vi "write_log_metadata.vi"(8 "error in (no error)":errorcluster, 10 "data":variant, 11 "pcfs_hdf5_log in":refnum<class "pcfs_hdf5_log.lvclass">) -> (0 "error out":errorcluster, 3 "pcfs_hdf5_log out":refnum<class "pcfs_hdf5_log.lvclass">)   [LabVIEW 2015, in "pcfs_hdf5_log.lvclass"]
uses:
  pcfs_hdf5_log.lvclass
  pcfs_settings.ctl
  Scan/scan_record.ctl
  Detector_Class/Picoquant/Hydraharp/hydraharp_panel/hpanel_acq_modes.ctl
  pcfs_hdf5_log.lvclass/pcfs_hdf5_log.ctl
  <vilib>/UPVI/lvhdf5/attribute.llb/LVH5A Operation.ctl
  <vilib>/UPVI/lvhdf5/attribute.llb/Simple H5Awrite (Variant).vi
  <vilib>/UPVI/lvhdf5/attribute.llb/Simple H5Awrite.xnode
  <vilib>/UPVI/lvhdf5/library.llb/HDF5 Ref.ctl
  Detector_Class/Picoquant/Hydraharp/hdf5_photon_record_logger/hdf5_photon_record_log.lvclass
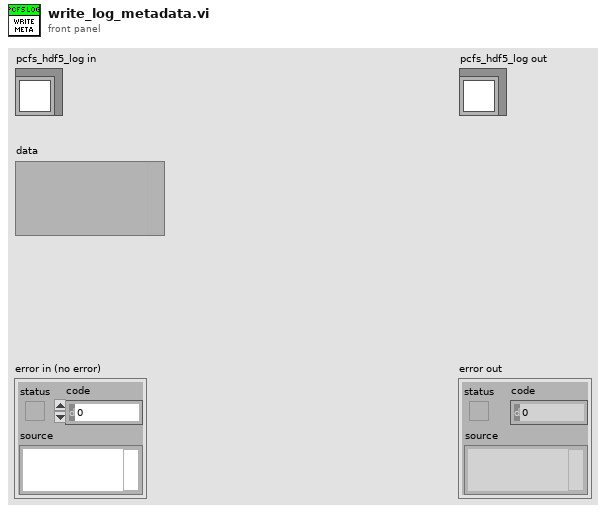
[diagram p1: front panel]
types:
  T1 = typedef "pcfs_settings.ctl" = cluster{"Center Pos. (mm)":dbl, "Increment (mm)":dbl, "Steps":dbl, "Dither Dist (nm)":dbl, "Dither Period (s)":dbl, "Cycles":dbl, "Record Type":T2, "Save Path":path, "Stage Number":enum16{"1", "2"}, "File Notes":string, "Mode":T3, "overwrite":bool, "custom_path":bool, "custom_positions":dbl[]}
  T2 = typedef "scan_record.ctl" = enum16{"hdf5", "legacy", "None"}
  T3 = typedef "hpanel_acq_modes.ctl" = u16
  T4 = typedef "LVH5A Operation.ctl" = enum16{"open", "replace", "create", "open or create", "create or replace", "create or replace with confirmation"}
  T5 = typedef "HDF5 Ref.ctl" = refnum<k1>
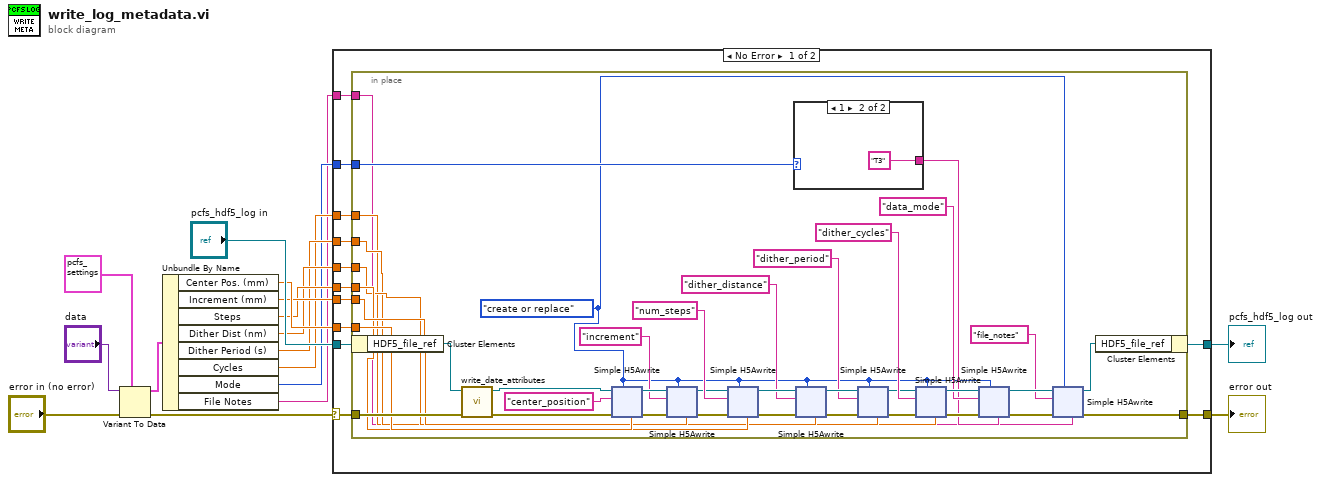
[diagram p0: block diagram]
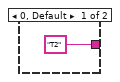
[diagram p2: hidden frame]
diagram:
  n1 = Variant To Data(error in="error in (no error)", type=T1 {"Center Pos. (mm)"=0.0, "Increment (mm)"=10.0, "Steps"=10.0, "Dither Dist (nm)"=10.0, "Dither Period (s)"=10.0, "Cycles"=10.0, "Record Type"=enum."hdf5", "Save Path"=path "C:/Users/bspoka/Desktop/test_pcfs", "Stage Number"=enum."1", "File Notes"="", "Mode"=2, "overwrite"=FALSE, "custom_path"=FALSE, "custom_positions"=[]} ("pcfs_settings"), Variant="data") -> (data=w11:T1, error out=w14:errorcluster)
  n2 = Unbundle By Name(w11) -> ("Center Pos. (mm)"=w10:dbl, "Increment (mm)"=w9:dbl, "Steps"=w8:dbl, "Dither Dist (nm)"=w7:dbl, "Dither Period (s)"=w6:dbl, "Cycles"=w5:dbl, "Mode"=w4:T3, "File Notes"=w3:string)
  n3 = case shown="No Error" w14 {
    selector: w14 -> [w27 w189]
    tunnel: "pcfs_hdf5_log in" -> [w28 w190]
    tunnel: w10 -> [w26 _]
    tunnel: w9 -> [w25 _]
    tunnel: w8 -> [w24 _]
    tunnel: w7 -> [w23 _]
    tunnel: w6 -> [w22 _]
    tunnel: w5 -> [w21 _]
    tunnel: w4 -> [w20 _]
    tunnel: w3 -> [w19 _]
    tunnel: [w18 w190] -> w2
    tunnel: [w17 w189] -> w1
    frame No Error {
      n4 = in-place {
        in-place-border: w27 -> [w65]
        in-place-border: w26 -> [w61]
        in-place-border: w25 -> [w57]
        in-place-border: w24 -> [w54]
        in-place-border: w23 -> [w49]
        in-place-border: w22 -> [w45]
        in-place-border: w21 -> [w42]
        in-place-border: w20 -> [w37]
        in-place-border: w19 -> [w32]
        in-place-border: [w29] -> w17
        w31 = LVH5A_Operation."create or replace" ("operation (open or create)")
        n5 = in-place-cluster #1(w28) -> ("HDF5_file_ref"=w66:T5)
        n6 = call "write_date_attributes.vi"("error in (no error)"=w65, "HDF5 Ref"=w66) -> ("error out"=w64:errorcluster, "HDF5 Ref out"=w63:T5)  [unwired: 8 in]
        n7 = xnode "Simple H5Awrite"("HDF5 Ref"=w63, "Name"="center_position", "error in (no error)"=w64, "operation (open or create)"=w31, "Value"=w61) -> ("HDF5 Ref out"=w59:T5, "error out"=w60:errorcluster)
        n8 = xnode "Simple H5Awrite"("HDF5 Ref"=w59, "Name"="increment", "error in (no error)"=w60, "operation (open or create)"=w31, "Value"=w57) -> ("HDF5 Ref out"=w55:T5, "error out"=w53:errorcluster)
        n9 = xnode "Simple H5Awrite"("HDF5 Ref"=w55, "Name"="num_steps", "error in (no error)"=w53, "operation (open or create)"=w31, "Value"=w54) -> ("HDF5 Ref out"=w51:T5, "error out"=w52:errorcluster)
        n10 = case shown="1" w37 {
          tunnel: ["T2" "T3"] -> w36
          frame 0, Default {
          }
          frame 1 {
          }
        }
        n11 = xnode "Simple H5Awrite"("HDF5 Ref"=w51, "Name"="dither_distance", "error in (no error)"=w52, "operation (open or create)"=w31, "Value"=w49) -> ("HDF5 Ref out"=w47:T5, "error out"=w48:errorcluster)
        n12 = xnode "Simple H5Awrite"("HDF5 Ref"=w47, "Name"="dither_period", "error in (no error)"=w48, "operation (open or create)"=w31, "Value"=w45) -> ("HDF5 Ref out"=w41:T5, "error out"=w44:errorcluster)
        n13 = xnode "Simple H5Awrite"("HDF5 Ref"=w41, "Name"="dither_cycles", "error in (no error)"=w44, "operation (open or create)"=w31, "Value"=w42) -> ("HDF5 Ref out"=w40:T5, "error out"=w39:errorcluster)
        n14 = xnode "Simple H5Awrite"("HDF5 Ref"=w40, "Name"="data_mode", "error in (no error)"=w39, "operation (open or create)"=w31, "Value"=w36) -> ("HDF5 Ref out"=w34:T5, "error out"=w35:errorcluster)
        n15 = xnode "Simple H5Awrite"("HDF5 Ref"=w34, "Name"="file_notes", "error in (no error)"=w35, "operation (open or create)"=w31, "Value"=w32) -> ("HDF5 Ref out"=w30:T5, "error out"=w29:errorcluster)
        n16 = in-place-cluster #1("HDF5_file_ref"=w30) -> (w18:refnum<class "pcfs_hdf5_log.lvclass">)
      }
    }
    frame Error {
    }
  }
  "error out" <- w1
  "pcfs_hdf5_log out" <- w2
